vi "SIM_CurrentOutput.vi"(9 "array":dbl[][](array[numeric]), 11 "Position 2":cluster{"X":dbl, "Y":dbl, "Z pen":dbl, "Z":dbl}) -> (3 "Current Out (pA)":dbl, 4 "Zread":dbl)   [LabVIEW 2019]
uses:
  <vilib>/ptbypt/NI_PtbyPt.lvlib
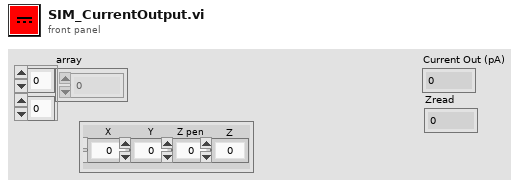
[diagram p1: front panel]
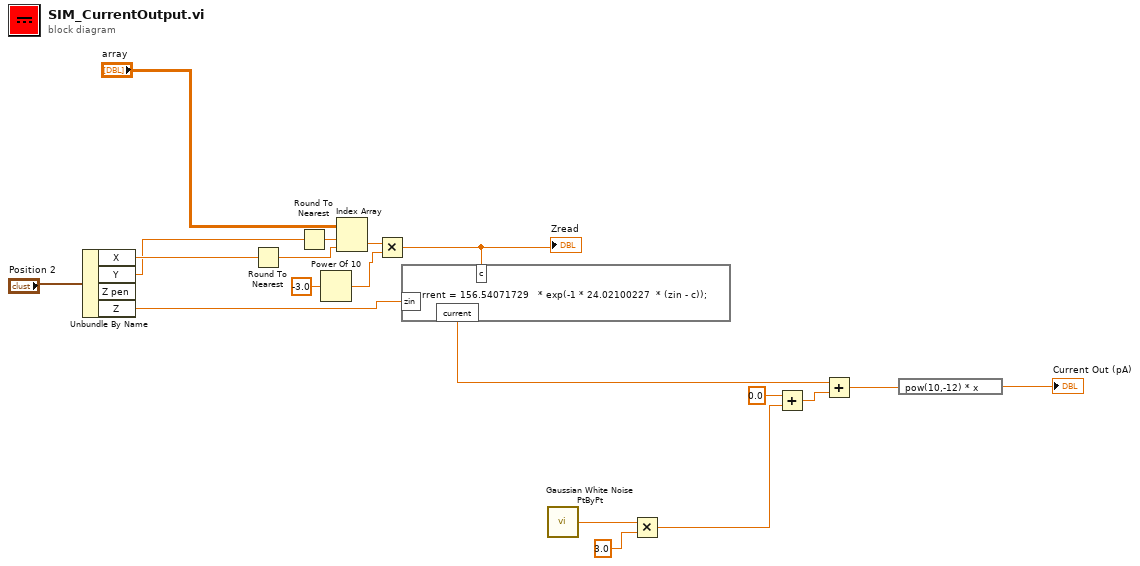
[diagram p0: block diagram]
diagram:
  n1 = Unbundle By Name("Position 2") -> ("X"=w5:dbl, "Y"=w4:dbl, "Z"=w3:dbl)  [unwired: 1 out]
  n2 = Round To Nearest(number=w5) -> (nearest integer value=w15:dbl)
  n3 = Round To Nearest(number=w4) -> (nearest integer value=w19:dbl)
  n4 = Power Of 10(x=-3.0) -> (10^x=w17:dbl)
  n5 = Index Array(array="array", index (row)=w19, index (col)=w15) -> (element=w14:dbl)
  n6 = Multiply(x=w14, y=w17) -> (x*y=w16:dbl)
  "Zread" <- w16
  n7 = formula code="current = 156.54071729   * exp(-1 * 24.02100227  * (zin - c));"("zin"=w3, "c"=w16) -> ("current"=w8:dbl)
  n8 = call <vilib>:"Gaussian White Noise PtByPt.vi"() -> ("Gaussian white noise"=w13:dbl)  [unwired: 3 in]
  n9 = Multiply(x=w13, y=3.0) -> (x*y=w10:dbl)
  n10 = Add(x=0.0, y=w10) -> (x+y=w11:dbl)
  n11 = Add(x=w8, y=w11) -> (x+y=w2:dbl)
  n12 = expression code="pow(10,-12) * x"(w2) -> (→"Current Out (pA)":dbl)
